vi "S2C_FORNAX_Proc_Close.vi"(8 "Error In":errorcluster) -> (0 "Error Out":errorcluster)   [LabVIEW 2015]
uses:
  S2C_FORNAX_Proc_Globals.vi
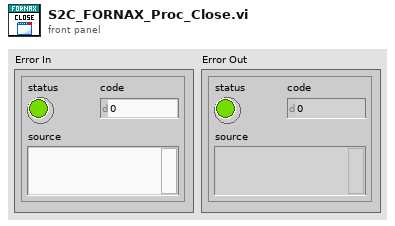
[diagram p1: front panel]
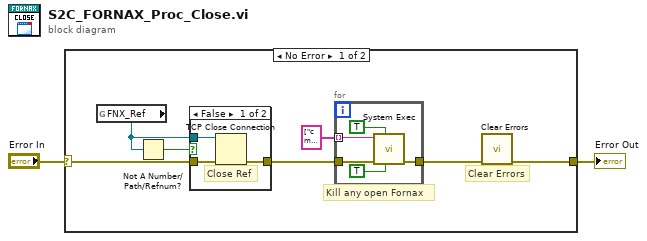
[diagram p0: block diagram]
diagram:
  n1 = case shown="No Error" "Error In" {
    selector: "Error In" -> [w9 w19]
    tunnel: [w3 w19] -> w1
    frame No Error {
      # "Clear Errors"
      # "Kill any open Fornax"
      n2 = global read "S2C_FORNAX_Proc_Globals.vi" "FNX_Ref"() -> (w6:refnum<k5>)
      n3 = Not A Number/Path/Refnum?(number/path/refnum=w6) -> (NaN/Path/Refnum?=w7:bool)
      n4 = case shown="False" w7 {
        tunnel: w9 -> [w12 w13]
        tunnel: w6 -> [w11 _]
        tunnel: [w10 w13] -> w5
        frame False {
          # "Close Ref"
          n5 = TCP Close Connection(connection ID=w11, error in (no error)=w12) -> (error out=w10:errorcluster)  [unwired: 1 in, 1 out]
        }
        frame True {
        }
      }
      n6 = for {
        tunnel: string[] ["cmd /c Taskkill /f /IM fornaxkirin.exe /T", "cmd /c Taskkill /f /IM fornax.exe /T", "cmd /c Taskkill /f /IM securefornax.exe /T"] -> [w16] mode=indexing
        tunnel: w5 -> [w15]
        tunnel: [w14] -> w4
        n7 = call <vilib>:"System Exec.vi"("run minimized? (F)"=TRUE, "wait until completion? (T)"=TRUE, "error in (no error)"=w15, "command line"=w16) -> ("error out"=w14:errorcluster)  [unwired: 4 in, 3 out]
      }
      n8 = call <vilib>:"Clear Errors.vi"("error in (no error)"=w4) -> ("error out"=w3:errorcluster)  [unwired: 5 in, 1 out]
    }
    frame Error {
    }
  }
  "Error Out" <- w1
